vi "Get Section.vi"(11 "Manufacturer Objects in":refnum<class "Manufacturer Objects.lvclass">) -> (2 "Section":string, 3 "Manufacturer Objects out":refnum<class "Manufacturer Objects.lvclass">)   [LabVIEW 2024, in "EDS.lvlib" / "Manufacturer Objects.lvclass"]
uses:
  Manufacturer Objects.lvclass
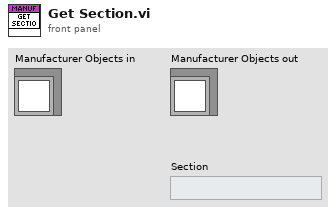
[diagram p1: front panel]
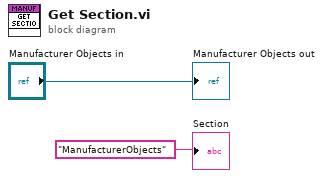
[diagram p0: block diagram]
diagram:
  "Manufacturer Objects out" <- "Manufacturer Objects in"
  "Section" <- "ManufacturerObjects" ("Section")
